vi "Can_Be_Package_Top_Level.vi"(8 "error in (no error)":errorcluster, 9 "AB_Source in":refnum<class "AB_Source.lvclass">, 11 "Build in":refnum<class "AB_PackedLibrary.lvclass">) -> (0 "error out":errorcluster, 2 "topLevel":bool, 3 "Build out":refnum<class "AB_PackedLibrary.lvclass">)   [LabVIEW 2020, in "AB_PackedLibrary.lvclass"]
uses:
  <vilib>/AppBuilder/AB_Classes/PackedLib/AB_PackedLibrary.lvclass
  <vilib>/AppBuilder/AB_Classes/Source/AB_Source.lvclass
  <vilib>/AppBuilder/AB_Classes/PackedLib/AB_PackedLibrary.lvclass/AB_PackedLibrary.ctl
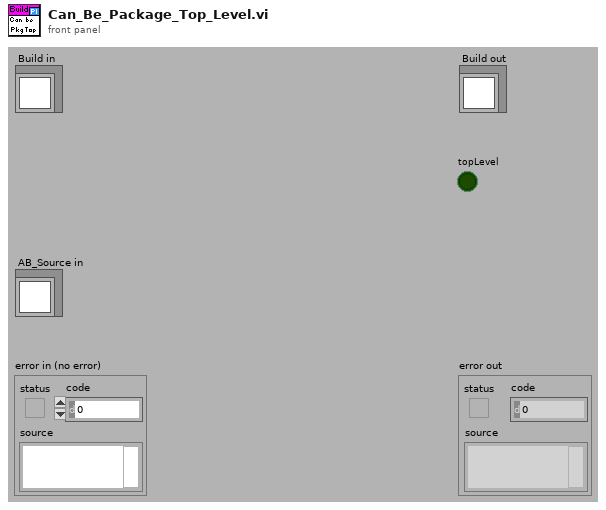
[diagram p1: front panel]
types:
  T1 = typedef "AB_Source.ctl" = cluster{"path":path, "itemID":string, "parentIndex":i32, "sourceInclusion":T2, "destinationIndex":i32, "properties":T3[], "newName":string, "lvfile":bool, "valid":bool, "eng_inBuild":bool, "eng_isNonVILink":bool, "Amalgamation":bool, "Amalgamation Piece":bool, "eng_delimitedName":string, "preventRename":bool}
  T2 = typedef "AB_Source_Inclusion.ctl" = enum16{"IncludeIfReferenced", "Include", "Exclude", "TopLevel"}
  T3 = typedef "AB_Source_Properties.ctl" = cluster{"sourcePropertyType":T4, "value":variant}
  T4 = typedef "AB_Source_Property_Type.ctl" = enum16{"Remove block diagram", "Remove front panel", "Password", "Window has title bar", "Show menu bar", "Show vertical scroll bar", "Show horizontal scroll bar", "Show toolbar", "Show Abort button", "Show fp when called", "Window behavior", "Allow user to close window", "Window run-time position", "Run when opened", "Allow debugging", "Auto error handling", "Generate guard code", "Use stack variables", "Expression folding", "Integer only", "Inline subVI"}
  T5 = enum32{"invalid scope", "public", "private", "protected", "community"}
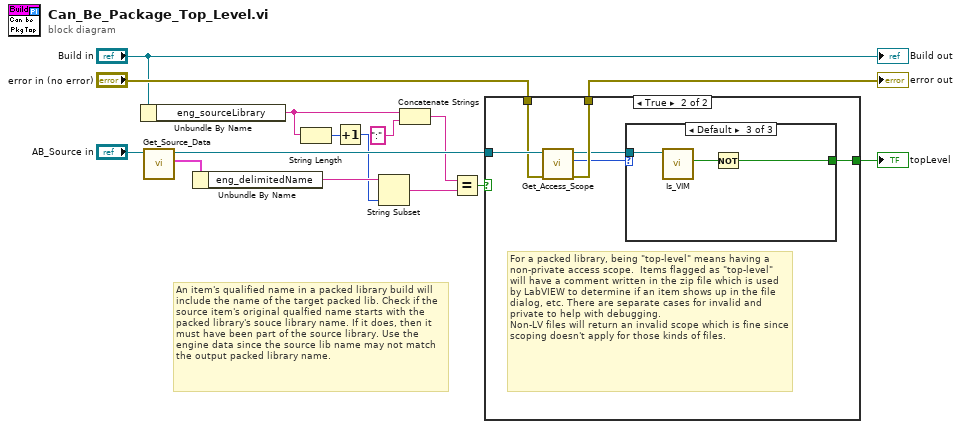
[diagram p0: block diagram]
diagram:
  # "An item's qualified name in a packed library build will include the name of the target packed lib. Check if the source item's original qualfied name starts with the packed library's souce library name. If it does, then it must have been part of the source library. Use the engine data since the source lib name may not match the output packed library name."
  n1 = Unbundle By Name("Build in") -> ("eng_sourceLibrary"=w5:string)
  n2 = call <vilib>:"Get_Source_Data.vi"("Class in"="AB_Source in") -> ("data"=w10:T1, "Class out"=w11:refnum<class "AB_Source.lvclass">)  [unwired: 8 in, 1 out]
  n3 = Unbundle By Name(w10) -> ("eng_delimitedName"=w8:string)
  n4 = String Length(string=w5) -> (length=w7:i32)
  n5 = Increment(x=w7) -> (x+1=w6:i32)
  n6 = String Subset(string=w8, length (rest)=w6) -> (substring=w2:string)  [unwired: 1 in]
  n7 = Concatenate Strings(w5, ":" ("string")) -> (w1:string)
  n8 = Equal?(x=w1, y=w2) -> (x = y?=w3:bool)
  n9 = case shown="True" w3 {
    tunnel: [_ w22] -> w15
    tunnel: w11 -> [_ w21]
    tunnel: "error in (no error)" -> [w16 w20]
    tunnel: [w16 w19] -> w13
    frame False {
      # "For a packed lib, items that were loose (not part of the source lib) are added to the source lib as part of the build process. Since these items were not originally in the source lib, do not make them visible from the packed lib."
    }
    frame True {
      # "For a packed library, being \"top-level\" means having a non-private access scope.  Items flagged as \"top-level\" will have a comment written in the zip file which is used by LabVIEW to determine if an item shows up in the file dialog, etc. There are separate cases for invalid and private to help with debugging.\nNon-LV files will return an invalid scope which is fine since scoping doesn't apply for those kinds of files."
      n10 = call-dynamic "Get_Access_Scope.vi"("error in (no error)"=w20, "AB_Source in"=w21) -> ("error out"=w19:errorcluster, "Source Scope"=w18:T5, "AB_Source out"=w17:refnum<class "AB_Source.lvclass">)  [unwired: 7 in]
      n11 = case shown="Default" w18 {
        tunnel: [_ _ w23] -> w22
        tunnel: w17 -> [_ _ w25]
        frame "invalid scope" {
        }
        frame "private" {
        }
        frame Default {
          n12 = call-dynamic "Is_VIM.vi"("AB_Source in"=w25) -> ("isVIM?"=w24:bool)  [unwired: 8 in, 2 out]
          n13 = Not(x=w24) -> (.not. x?=w23:bool)
        }
      }
    }
  }
  "error out" <- w13
  "topLevel" <- w15
  "Build out" <- "Build in"
